vi "Get Focus Rects.vi"(8 "error in (no error)":errorcluster, 11 "Scalable Border in":refnum<class "Scalable Border.lvclass">) -> (0 "error out":errorcluster, 2 "Focus Rects":T1(array[cluster]), 3 "Scalable Border out":refnum<class "Scalable Border.lvclass">)   [LabVIEW 2015, in "Scalable Border.lvclass"]
uses:
  Scalable Border.lvclass
  Scalable Border.lvclass/Scalable Border.ctl
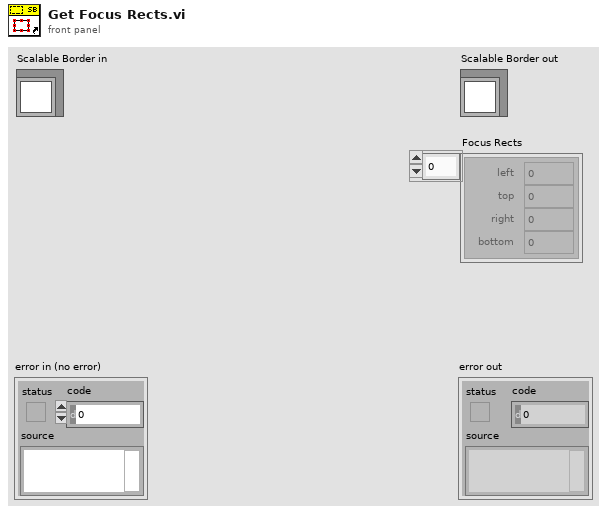
[diagram p1: front panel]
types:
  T1 = cluster{"left":i16, "top":i16, "right":i16, "bottom":i16}[]
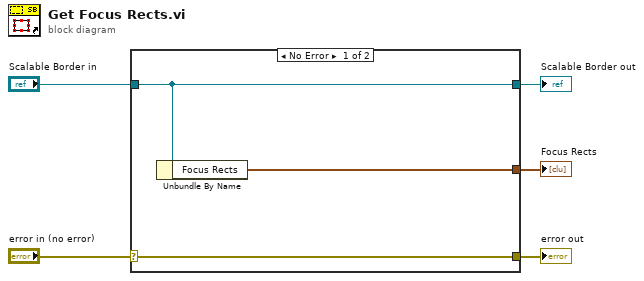
[diagram p0: block diagram]
diagram:
  n1 = case shown="No Error" "error in (no error)" {
    selector: "error in (no error)" -> [w8 w9]
    tunnel: [w8 w9] -> w4
    tunnel: [w7 w10] -> w2
    tunnel: "Scalable Border in" -> [w7 w10]
    tunnel: [w6 _] -> w1
    frame No Error {
      n2 = Unbundle By Name(w7) -> ("Focus Rects"=w6:T1)
    }
    frame Error {
    }
  }
  "error out" <- w4
  "Scalable Border out" <- w2
  "Focus Rects" <- w1
